vi "VI Default Control.vi"(8 "error in":errorcluster, 11 "VI Reference in":refnum<vi>) -> (0 "error out":errorcluster, 3 "VI Reference out":refnum<vi>)   [LabVIEW 2018]
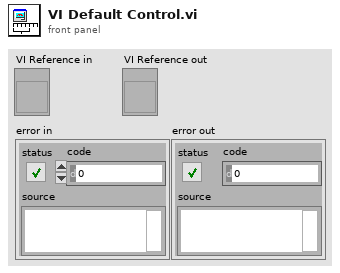
[diagram p1: front panel]
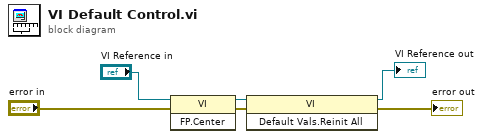
[diagram p0: block diagram]
diagram:
  n1 = invoke class="VI" method="FP.Center"(reference="VI Reference in", error in="error in") -> (reference out=w5:refnum<vi>, error out=w6:errorcluster)  [unwired: 1 in, 1 out]
  n2 = invoke class="VI" method="Default Vals.Reinit All"(reference=w5, error in=w6) -> (reference out=→"VI Reference out":refnum<vi>, error out=→"error out":errorcluster)  [unwired: 1 in, 1 out]
